vi "Exemple_Impute_KNNImputer.vi"() -> ()   [LabVIEW 2020]
uses:
  Objet/6 - Datasets Transformation/6.4 - Imputation of missing values/KNNImputer/KNNImputer.lvclass
panel:
  in  "KNNImputer":T1={"missing_values"="nan", "n_neighbors"=5, "weights"="uniform", "metric"="nan_euclidean", "copy"=TRUE, "add_indicator"=FALSE}
  out "Data":T2
  out "error out":errorcluster caption="sortie d'erreur"
  in  "y":string[][](array[string])
  in  "X":string[][](array[string])=[["1", "2", "nan"], ["3", "4", "3"], ["nan", "6", "5"]]
  in  "error in":errorcluster caption="entrée d'erreur"
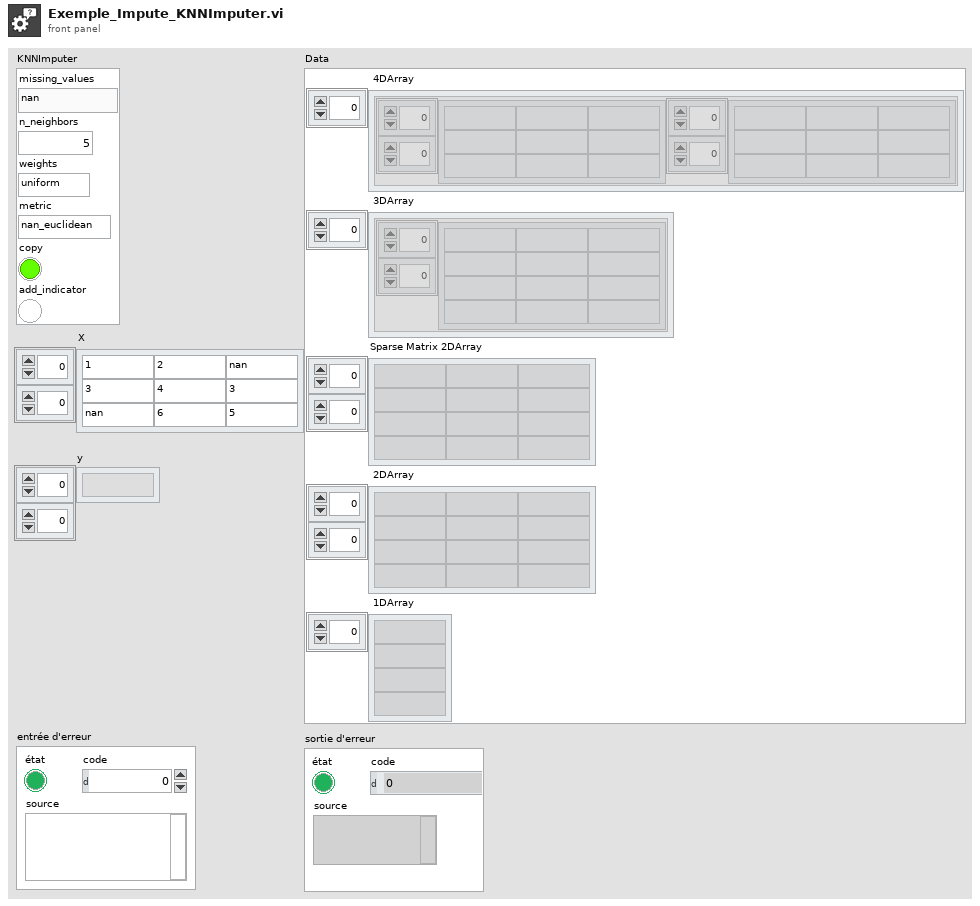
[diagram p1: front panel]
types:
  T1 = cluster{"missing_values":string, "n_neighbors":i32, "weights":string, "metric":string, "copy":bool, "add_indicator":bool}
  T2 = cluster{" 4DArray":cluster{"1":string[][], "2":string[][]}[], " 3DArray":cluster{"Tableau":string[][]}[], "Sparse Matrix 2DArray":string[][], " 2DArray":string[][], " 1DArray":string[]}
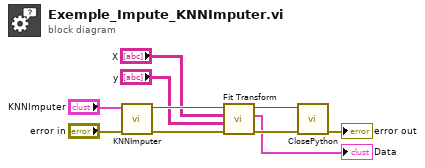
[diagram p0: block diagram]
diagram:
  n1 = call "KNNImputer.vi"("error in"="error in", "KNNImputer"="KNNImputer") -> ("error out"=w8:errorcluster, "KNNImputer.lvclass"=w7:refnum<class "KNNImputer.lvclass">)  [unwired: 8 in]
  n2 = call-dynamic "Fit Transform.vi"("error in (no error)"=w8, "y"="y", "X"="X", "KNNImputer.lvclass"=w7) -> ("error out"=w3:errorcluster, "Data"=→"Data":T2, "KNNImputer.lvclass"=w4:refnum<class "KNNImputer.lvclass">)  [unwired: 5 in]
  n3 = call-dynamic "ClosePython.vi"("error in (no error)"=w3, "Scikit-learn en entrée"=w4) -> ("error out"=→"error out":errorcluster)  [unwired: 8 in, 1 out]
